vi "Cal10-WriteOutCurrentSetup.vi"(8 "poly fit order":i32=2 caption="Polynomial\nOrder" min=1 max=4 step=1, 11 "CalibrationPath":path) -> (3 "String":string)   [LabVIEW 2021]
uses:
  Anemometry Sub Vis/File/Setup_Filetype.ctl
  Anemometry Sub Vis/Globals/Calib_global.vi
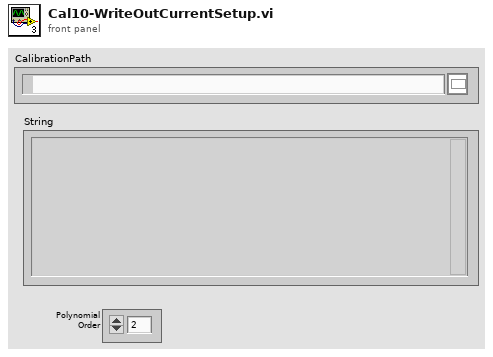
[diagram p1: front panel]
types:
  T1 = typedef "Setup_Filetype.ctl" = enum16{"Measurement Setups", "Calibration Setups", "General", "Results File Plotter Setups", "Speed Calib Tweaks"}
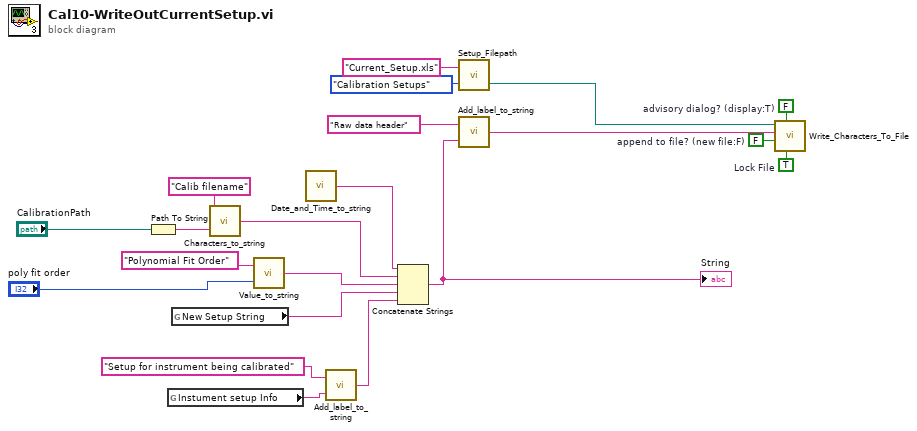
[diagram p0: block diagram]
diagram:
  w16 = TRUE  # Lock File
  w11 = FALSE  # advisory dialog? (display:T)
  w10 = FALSE  # append to file? (new file:F)
  n1 = Path To String(path="CalibrationPath") -> (string=w15:string)
  n2 = global read "Calib_global.vi" "Instument setup Info"() -> (w6:string)
  n3 = global read "Calib_global.vi" "New Setup String"() -> (w14:string)
  n4 = call "Characters_to_string.vi"("Characters to write"=w15, "Label for characters"="Calib filename") -> ("Output string"=w7:string)  [unwired: 1 in]
  n5 = call "Value_to_string.vi"("Value"="poly fit order", "Label for value"="Polynomial Fit Order") -> ("Output string"=w1:string)  [unwired: 1 in]
  n6 = call "Date_and_Time_to_string.vi"() -> ("Date and time (spreadsheet)"=w8:string)  [unwired: 4 in, 1 out]
  n7 = call "Add_label_to_string.vi"("String to write"=w6, "File Label"="Setup for instrument being calibrated") -> ("Output string"=w4:string)
  n8 = Concatenate Strings(w8, w7, w1, w14, w4) -> (w18:string)
  "String" <- w18
  n9 = call "Setup_Filepath.vi"("Setup File Type"=Setup_Filetype."Calibration Setups", "Filename in"="Current_Setup.xls") -> ("Filename Out"=w21:path)  [unwired: 1 out]
  n10 = call "Add_label_to_string.vi"("String to write"=w18, "File Label"="Raw data header") -> ("Output string"=w13:string)
  n11 = call "Write_Characters_To_File.vi"("file path (dialog if empty)"=w21, "advisory dialog? (display:T)"=w11, "character string"=w13, "append to file? (new file:F)"=w10, "Lock File"=w16) -> ()  [unwired: 4 out]
